vi "DashboardGetvi.vi"(9 "Joystick 1":T1) -> ()   [LabVIEW 2018]
uses:
  <vilib>/Rock Robotics/WPI/Joystick/WPI_JoystickDevRef.ctl
  <vilib>/Rock Robotics/WPI/Joystick/WPI_JoystickDeviceEnum.ctl
  <vilib>/Rock Robotics/Network Tables/NT Read Boolean.vi
  <vilib>/Rock Robotics/Network Tables/NT Read Number.vi
  Inputs_DriverStation.vi
  RobotStates.vi
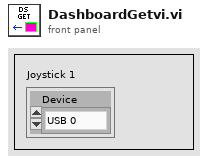
[diagram p1: front panel]
types:
  T1 = typedef "WPI_JoystickDevRef.ctl" = cluster{"Device":T2}
  T2 = typedef "WPI_JoystickDeviceEnum.ctl" = enum16{"USB 0", "USB 1", "USB 2", "USB 3", "USB 4", "USB 5"}
  T3 = cluster{"Boolean":bool, "Boolean":bool, "Boolean":bool, "Boolean":bool, "Boolean":bool, "Boolean":bool, "Boolean":bool, "Boolean":bool, "Boolean":bool, "Boolean":bool, "Boolean":bool, "Boolean":bool, "Boolean":bool, "Boolean":bool}
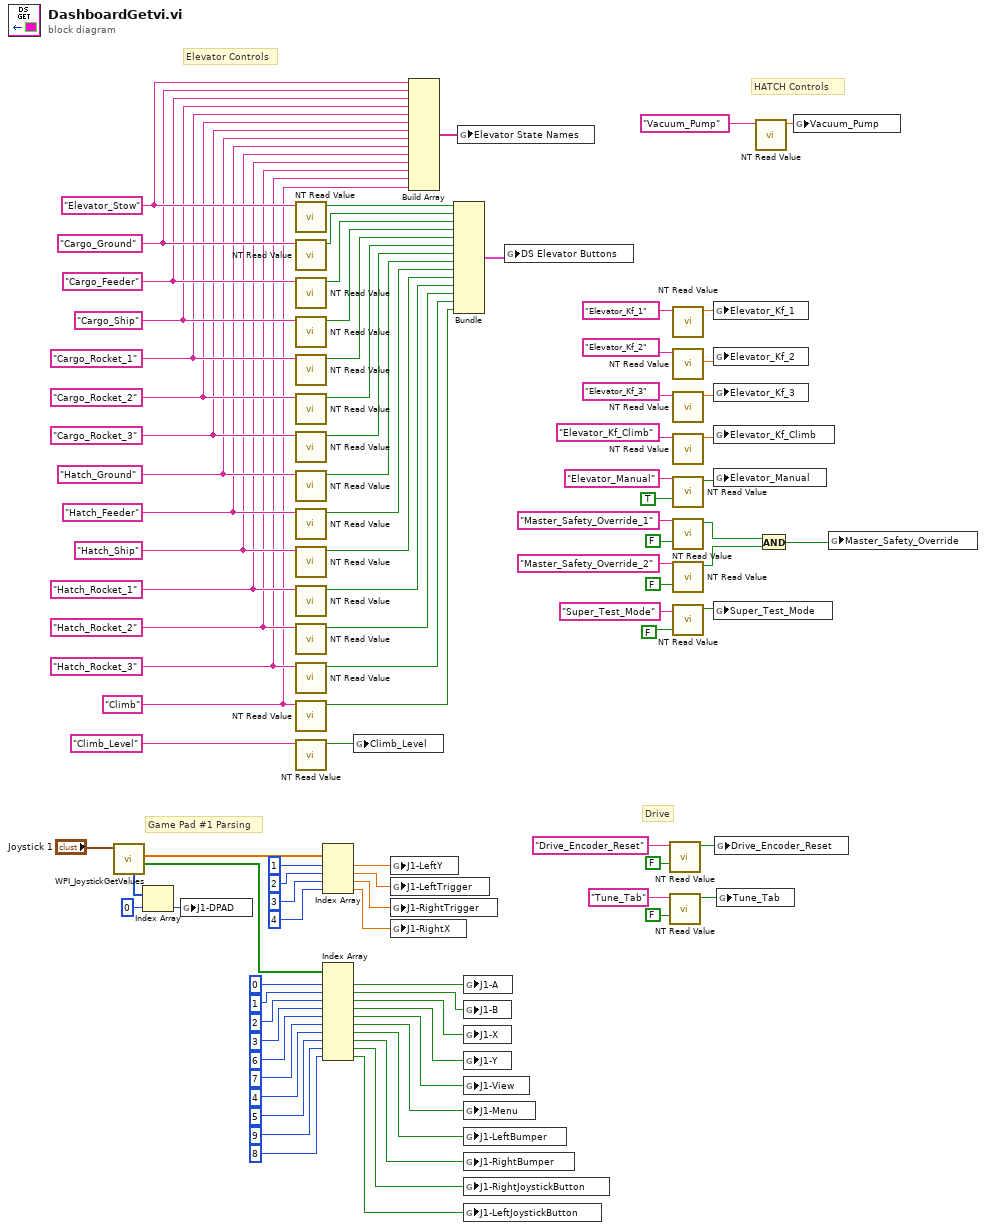
[diagram p0: block diagram]
diagram:
  w24 = "Climb" ("refnum name")
  w32 = "Hatch_Rocket_3" ("refnum name")
  w33 = "Hatch_Rocket_2" ("refnum name")
  w34 = "Hatch_Rocket_1" ("refnum name")
  w35 = "Hatch_Ship" ("refnum name")
  w36 = "Hatch_Feeder" ("refnum name")
  w37 = "Hatch_Ground" ("refnum name")
  w81 = "Cargo_Rocket_3" ("refnum name")
  w82 = "Cargo_Rocket_2" ("refnum name")
  w83 = "Cargo_Rocket_1" ("refnum name")
  w84 = "Cargo_Ship" ("refnum name")
  w90 = "Cargo_Feeder" ("refnum name")
  w91 = "Cargo_Ground" ("refnum name")
  w92 = "Elevator_Stow" ("refnum name")
  # "Drive"
  # "HATCH Controls"
  # "Game Pad #1 Parsing"
  # "Elevator Controls"
  n1 = call <vilib>:"WPI_JoystickGetValues.vi"("JoystickDevRef"="Joystick 1") -> ("Buttons"=w72:bool[], "Axes"=w71:dbl[], "POVs"=w68:i16[])  [unwired: 6 in, 2 out]
  n2 = Index Array(array=w68, index=0) -> (element=w65:i16)
  n3 = global write "Inputs_DriverStation.vi" "J1-DPAD"(w65) -> ()
  n4 = call-poly <vilib>:"NT Read Value.vi"("Name"=w92) -> ("Boolean"=w95:bool)  [unwired: 9 in, 1 out]
  n5 = call-poly <vilib>:"NT Read Value.vi"("Name"=w91) -> ("Boolean"=w94:bool)  [unwired: 9 in, 1 out]
  n6 = call-poly <vilib>:"NT Read Value.vi"("Name"=w90) -> ("Boolean"=w93:bool)  [unwired: 9 in, 1 out]
  n7 = call-poly <vilib>:"NT Read Value.vi"("Name"=w84) -> ("Boolean"=w88:bool)  [unwired: 9 in, 1 out]
  n8 = call-poly <vilib>:"NT Read Value.vi"("Name"=w83) -> ("Boolean"=w87:bool)  [unwired: 9 in, 1 out]
  n9 = call-poly <vilib>:"NT Read Value.vi"("Name"=w82) -> ("Boolean"=w86:bool)  [unwired: 9 in, 1 out]
  n10 = call-poly <vilib>:"NT Read Value.vi"("Name"=w81) -> ("Boolean"=w85:bool)  [unwired: 9 in, 1 out]
  n11 = call-poly <vilib>:"NT Read Value.vi"("Name"=w37) -> ("Boolean"=w44:bool)  [unwired: 9 in, 1 out]
  n12 = call-poly <vilib>:"NT Read Value.vi"("Name"=w36) -> ("Boolean"=w43:bool)  [unwired: 9 in, 1 out]
  n13 = call-poly <vilib>:"NT Read Value.vi"("Name"=w35) -> ("Boolean"=w42:bool)  [unwired: 9 in, 1 out]
  n14 = call-poly <vilib>:"NT Read Value.vi"("Name"=w34) -> ("Boolean"=w41:bool)  [unwired: 9 in, 1 out]
  n15 = call-poly <vilib>:"NT Read Value.vi"("Name"=w33) -> ("Boolean"=w40:bool)  [unwired: 9 in, 1 out]
  n16 = call-poly <vilib>:"NT Read Value.vi"("Name"=w32) -> ("Boolean"=w39:bool)  [unwired: 9 in, 1 out]
  n17 = call-poly <vilib>:"NT Read Value.vi"("Name"=w24) -> ("Boolean"=w23:bool)  [unwired: 9 in, 1 out]
  n18 = call-poly <vilib>:"NT Read Value.vi"("Name"="Climb_Level" ("refnum name")) -> ("Boolean"=w21:bool)  [unwired: 9 in, 1 out]
  n19 = Index Array(array=w71, index #1=1 ("index"), index #2=2 ("index"), index #3=3 ("index"), index #4=4 ("index")) -> (element #1=w58:dbl, element #2=w59:dbl, element #3=w60:dbl, element #4=w57:dbl)
  n20 = Index Array(array=w72, index #1=0 ("index"), index #2=1 ("index"), index #3=2 ("index"), index #4=3 ("index"), index #5=6 ("index"), index #6=7 ("index"), index #7=4 ("index"), index #8=5 ("index"), index #9=9 ("index"), index #10=8 ("index")) -> (element #1=w64:bool, element #2=w63:bool, element #3=w62:bool, element #4=w61:bool, element #5=w19:bool, element #6=w15:bool, element #7=w12:bool, element #8=w11:bool, element #9=w9:bool, element #10=w4:bool)
  n21 = global write "Inputs_DriverStation.vi" "Climb_Level"(w21) -> ()
  n22 = global write "Inputs_DriverStation.vi" "J1-LeftY"(w58) -> ()
  n23 = global write "Inputs_DriverStation.vi" "J1-LeftTrigger"(w59) -> ()
  n24 = global write "Inputs_DriverStation.vi" "J1-RightTrigger"(w60) -> ()
  n25 = global write "Inputs_DriverStation.vi" "J1-RightX"(w57) -> ()
  n26 = Build Array(w92, w91, w90, w84, w83, w82, w81, w37, w36, w35, w34, w33, w32, w24) -> (w89:string[])
  n27 = Bundle("Boolean"=w95, "Boolean"=w94, "Boolean"=w93, "Boolean"=w88, "Boolean"=w87, "Boolean"=w86, "Boolean"=w85, "Boolean"=w44, "Boolean"=w43, "Boolean"=w42, "Boolean"=w41, "Boolean"=w40, "Boolean"=w39, "Boolean"=w23) -> (w38:T3)  [unwired: 1 in]
  n28 = global write "RobotStates.vi" "Elevator State Names"(w89) -> ()
  n29 = global write "Inputs_DriverStation.vi" "J1-A"(w64) -> ()
  n30 = global write "Inputs_DriverStation.vi" "J1-B"(w63) -> ()
  n31 = global write "Inputs_DriverStation.vi" "J1-X"(w62) -> ()
  n32 = global write "Inputs_DriverStation.vi" "J1-Y"(w61) -> ()
  n33 = global write "Inputs_DriverStation.vi" "J1-View"(w19) -> ()
  n34 = global write "Inputs_DriverStation.vi" "J1-Menu"(w15) -> ()
  n35 = global write "Inputs_DriverStation.vi" "J1-LeftBumper"(w12) -> ()
  n36 = global write "Inputs_DriverStation.vi" "J1-RightBumper"(w11) -> ()
  n37 = global write "Inputs_DriverStation.vi" "J1-RightJoystickButton"(w9) -> ()
  n38 = global write "Inputs_DriverStation.vi" "J1-LeftJoystickButton"(w4) -> ()
  n39 = global write "Inputs_DriverStation.vi" "DS Elevator Buttons"(w38) -> ()
  n40 = call-poly <vilib>:"NT Read Value.vi"("Default Value"=FALSE, "Name"="Drive_Encoder_Reset" ("refnum name")) -> ("Boolean"=w45:bool)  [unwired: 8 in, 1 out]
  n41 = call-poly <vilib>:"NT Read Value.vi"("Default Value"=FALSE, "Name"="Tune_Tab" ("refnum name")) -> ("Boolean"=w6:bool)  [unwired: 8 in, 1 out]
  n42 = call-poly <vilib>:"NT Read Value.vi"("Name"="Elevator_Kf_1" ("refnum name")) -> ("Numeric"=w79:dbl)  [unwired: 9 in, 1 out]
  n43 = call-poly <vilib>:"NT Read Value.vi"("Name"="Elevator_Kf_2" ("refnum name")) -> ("Numeric"=w52:dbl)  [unwired: 9 in, 1 out]
  n44 = call-poly <vilib>:"NT Read Value.vi"("Name"="Elevator_Kf_3" ("refnum name")) -> ("Numeric"=w50:dbl)  [unwired: 9 in, 1 out]
  n45 = call-poly <vilib>:"NT Read Value.vi"("Name"="Elevator_Kf_Climb" ("refnum name")) -> ("Numeric"=w17:dbl)  [unwired: 9 in, 1 out]
  n46 = call-poly <vilib>:"NT Read Value.vi"("Default Value"=TRUE, "Name"="Elevator_Manual" ("refnum name")) -> ("Boolean"=w55:bool)  [unwired: 8 in, 1 out]
  n47 = call-poly <vilib>:"NT Read Value.vi"("Default Value"=FALSE, "Name"="Master_Safety_Override_1" ("refnum name")) -> ("Boolean"=w27:bool)  [unwired: 8 in, 1 out]
  n48 = call-poly <vilib>:"NT Read Value.vi"("Default Value"=FALSE, "Name"="Master_Safety_Override_2" ("refnum name")) -> ("Boolean"=w26:bool)  [unwired: 8 in, 1 out]
  n49 = call-poly <vilib>:"NT Read Value.vi"("Default Value"=FALSE, "Name"="Super_Test_Mode" ("refnum name")) -> ("Boolean"=w2:bool)  [unwired: 8 in, 1 out]
  n50 = global write "Inputs_DriverStation.vi" "Elevator_Kf_1"(w79) -> ()
  n51 = global write "Inputs_DriverStation.vi" "Elevator_Kf_2"(w52) -> ()
  n52 = global write "Inputs_DriverStation.vi" "Elevator_Kf_3"(w50) -> ()
  n53 = global write "Inputs_DriverStation.vi" "Elevator_Kf_Climb"(w17) -> ()
  n54 = global write "Inputs_DriverStation.vi" "Elevator_Manual"(w55) -> ()
  n55 = global write "Inputs_DriverStation.vi" "Super_Test_Mode"(w2) -> ()
  n56 = global write "Inputs_DriverStation.vi" "Drive_Encoder_Reset"(w45) -> ()
  n57 = global write "Inputs_DriverStation.vi" "Tune_Tab"(w6) -> ()
  n58 = call-poly <vilib>:"NT Read Value.vi"("Name"="Vacuum_Pump" ("refnum name")) -> ("Numeric"=w48:dbl)  [unwired: 9 in, 1 out]
  n59 = And(x=w27, y=w26) -> (x .and. y?=w25:bool)
  n60 = global write "Inputs_DriverStation.vi" "Vacuum_Pump"(w48) -> ()
  n61 = global write "Inputs_DriverStation.vi" "Master_Safety_Override"(w25) -> ()
